vi "Reset.vi"(8 "error in (no error)":errorcluster, 11 "VISA resource name":refnum<visa-resource-name>) -> (0 "error out":errorcluster, 3 "VISA resource name out":refnum<visa-resource-name>)   [LabVIEW 2015, in "Fluke 8808.lvlib"]
doc: "Resets the instrument and then sends a set of default setup commands to the instrument."
uses:
  <instrlib>/Fluke 8808/Fluke 8808.lvlib
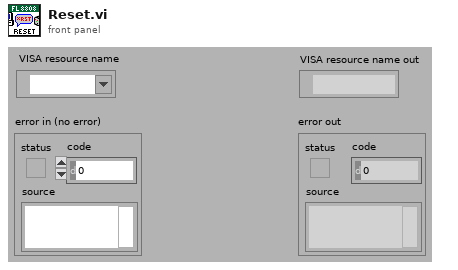
[diagram p1: front panel]
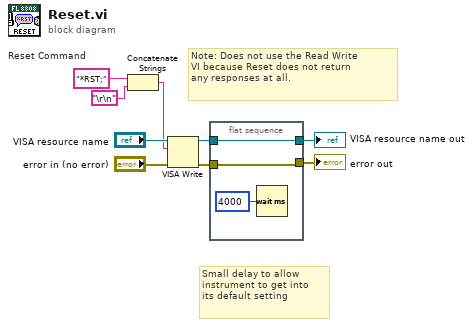
[diagram p0: block diagram]
diagram:
  w7 = "*RST;"  # Reset Command
  # "Note: Does not use the Read Write\nVI because Reset does not return\nany responses at all."
  # "Small delay to allow\ninstrument to get into\nits default setting"
  n1 = Concatenate Strings(w7, "\r\n") -> (w5:string)
  n2 = VISA Write(VISA resource name="VISA resource name", write buffer=w5, error in (no error)="error in (no error)") -> (VISA resource name out=w4:refnum<visa-resource-name>, error out=w1:errorcluster)  [unwired: 1 out]
  n3 = flat-sequence {
    tunnel: w4 -> [w12]
    tunnel: [w12] -> w3
    tunnel: [w11] -> w2
    tunnel: w1 -> [w11]
    frame #0 {
      n4 = Wait (ms)(milliseconds to wait=u32 4000) -> ()  [unwired: 1 out]
    }
  }
  "error out" <- w2
  "VISA resource name out" <- w3
